vi "CoreQueuesCreate.vi"() -> (3 "Cluster":T1)   [LabVIEW 2024]
uses:
  <vilib>/vision/Image Controls.llb/IMAQ Image.ctl
  vision/#QueueEnum.ctl
  #CoreQueues.ctl
  GUI/#GuiEnum.ctl
  GUI/#GuiQueueElement.ctl
  Correlation/#CorrelationQueueElement.ctl
  vision/#VideoQueueElement.ctl
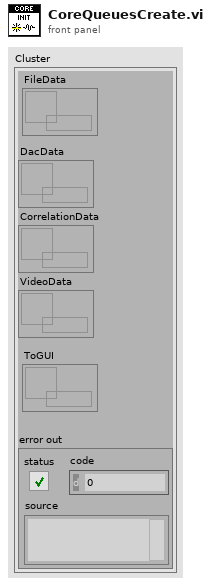
[diagram p1: front panel]
types:
  T1 = typedef "#CoreQueues.ctl" = cluster{"DacData":refnum<queue>, "CorrelationData":refnum<queue>, "VideoData":refnum<queue>, "error out":errorcluster, "ToGUI":refnum<queue>, "FileData":refnum<queue>}
  T2 = typedef "#CorrelationQueueElement.ctl" = cluster{"Enum":T3, "t0":timestamp, dbl[]}
  T3 = typedef "#QueueEnum.ctl" = enum16{"Ant", "Video"}
  T4 = typedef "#VideoQueueElement.ctl" = cluster{"Image Out":T5, "current time":timestamp}
  T5 = typedef "IMAQ Image.ctl" = refnum<image>
  T6 = typedef "#GuiQueueElement.ctl" = cluster{"Enum":T7, "Variant":variant}
  T7 = typedef "#GuiEnum.ctl" = enum16{"AudioData", "VisionDistances", "DacDistances", "CorrelationDistances", "Video", "FPS"}
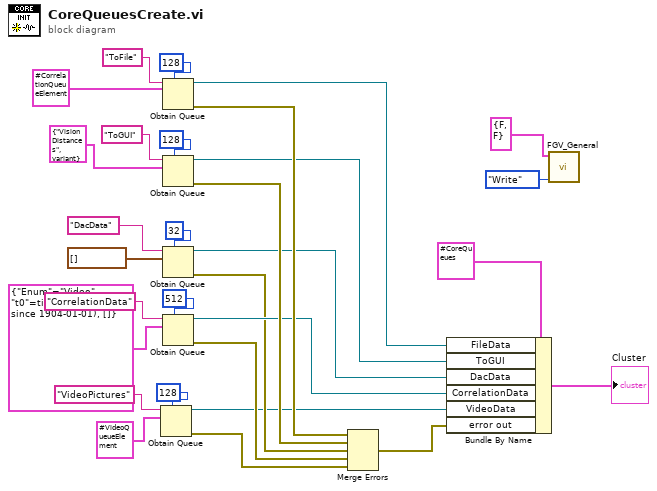
[diagram p0: block diagram]
diagram:
  n1 = Obtain Queue(max queue size (-1, unlimited)=128, name (unnamed)="VideoPictures", element data type=T4 {"Image Out"=refnum, "current time"=timestamp(0 s since 1904-01-01)}) -> (queue out=w20:refnum<queue>, error out=w21:errorcluster)  [unwired: 2 in, 1 out]
  n2 = Obtain Queue(max queue size (-1, unlimited)=128, name (unnamed)="ToFile", element data type=T2 {"Enum"=enum."Video", "t0"=timestamp(0 s since 1904-01-01), []}) -> (queue out=w30:refnum<queue>, error out=w29:errorcluster)  [unwired: 2 in, 1 out]
  n3 = Obtain Queue(max queue size (-1, unlimited)=128, name (unnamed)="ToGUI", element data type=T6 {"Enum"=enum."VisionDistances", "Variant"=variant}) -> (queue out=w28:refnum<queue>, error out=w27:errorcluster)  [unwired: 2 in, 1 out]
  n4 = Obtain Queue(max queue size (-1, unlimited)=32, name (unnamed)="DacData", element data type=waveform(dbl)[] [] ("data")) -> (queue out=w26:refnum<queue>, error out=w23:errorcluster)  [unwired: 2 in, 1 out]
  n5 = Obtain Queue(max queue size (-1, unlimited)=512, name (unnamed)="CorrelationData", element data type=T2 {"Enum"=enum."Video", "t0"=timestamp(0 s since 1904-01-01), []}) -> (queue out=w25:refnum<queue>, error out=w22:errorcluster)  [unwired: 2 in, 1 out]
  n6 = Merge Errors(w29, w27, w23, w22, w21) -> (w24:errorcluster)
  n7 = Bundle By Name(cluster=T1 {"DacData"=refnum, "CorrelationData"=refnum, "VideoData"=refnum, "error out"={"status"=FALSE, "code"=0, "source"=""}, "ToGUI"=refnum, "FileData"=refnum}, "FileData"=w30, "ToGUI"=w28, "DacData"=w26, "CorrelationData"=w25, "VideoData"=w20, "error out"=w24) -> (→"Cluster":T1)
  n8 = call "FGV_General.vi"("Type"=enum16{"Read", "Write"}."Write", "GeneralControl"=cluster{"StartButton":bool, "StopButton":bool} {"StartButton"=FALSE, "StopButton"=FALSE}) -> ()  [unwired: 9 in, 1 out]
